vi "_FPGA_EventHandler.vi"(0 "LoadNextEvent_strobe":bool=TRUE, 7 "Reset_strobe":bool) -> (10 "Index+1?":u8, 12 "End?":bool, 13 "NewEvent_strobe?":bool, 14 "EventCode":u8, 15 "Param 1":u64, 16 "Param 2":u64, 17 "Param 3":u64, 18 "Param 4":u64, 19 "Param 5":u64)   [LabVIEW 2018]
uses:
  <instrlib>/_niInstr/Basic Elements/v1/FPGA/niInstr Basic Elements v1 FPGA.lvlib
  <instrlib>/_niInstr/Basic Elements/v1/FPGA/Private/Count Up U8.vi
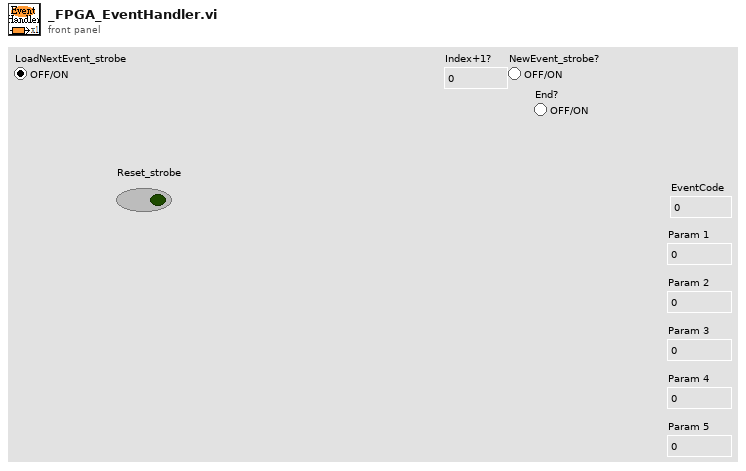
[diagram p1: front panel]
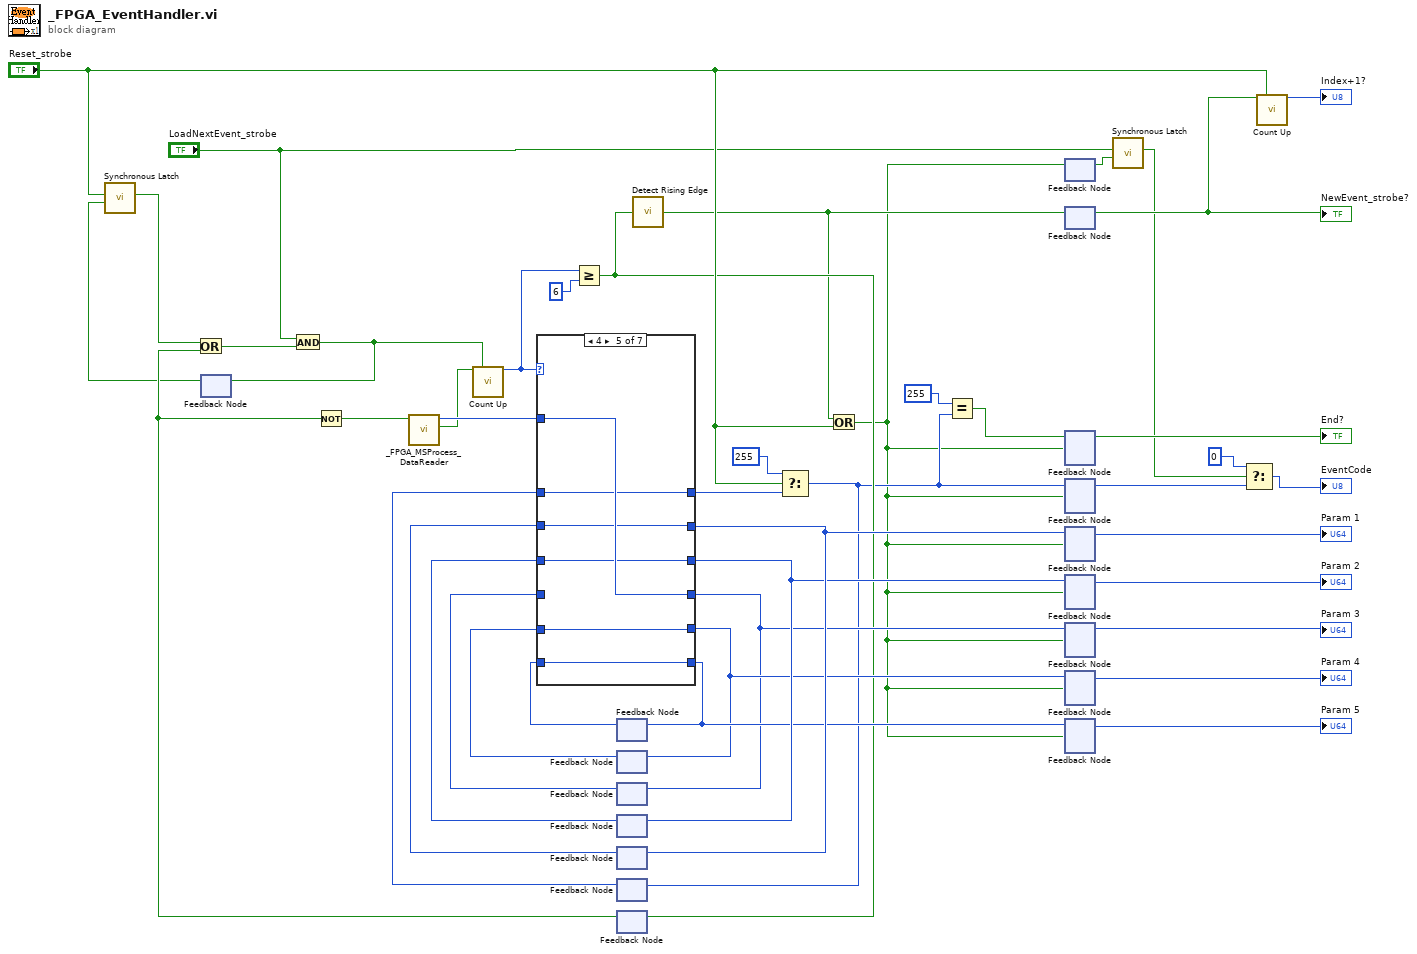
[diagram p0: block diagram]
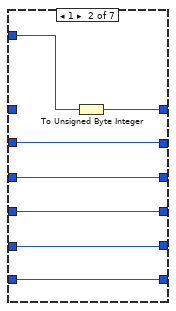
[diagram p3: hidden frame]
diagram:
  n1 = feedback #1() -> (w15:bool)  [unwired: 1 in]
  n2 = call <instrlib>:"Synchronous Latch.vi"("clear"=w15, "set"="Reset_strobe") -> ("out"=w14:bool)  [unwired: 9 in]
  n3 = feedback #2() -> (w41:u64)  [unwired: 1 in]
  n4 = feedback #3() -> (w40:u64)  [unwired: 1 in]
  n5 = feedback #4() -> (w39:u64)  [unwired: 1 in]
  n6 = feedback #5() -> (w32:u64)  [unwired: 1 in]
  n7 = feedback #6() -> (w33:u64)  [unwired: 1 in]
  n8 = feedback #7() -> (w34:u8)  [unwired: 1 in]
  n9 = feedback #8() -> (w20:bool)  [unwired: 1 in]
  n10 = Or(x=w14, y=w20) -> (x .or. y?=w16:bool)
  n11 = And(x="LoadNextEvent_strobe", y=w16) -> (x .and. y?=w8:bool)
  n12 = feedback-in #1(w8) -> ()
  n13 = Not(x=w20) -> (.not. x?=w36:bool)
  n14 = call "_FPGA_MSProcess_DataReader.vi"("Read"=w36) -> ("new value"=w42:bool, "Element"=w43:u64)  [unwired: 9 in]
  n15 = call-poly <instrlib>:"Count Up.vi"("increment"=w42, "reset"=w8) -> ("count out"=w38:u8)  [unwired: 13 in]
  n16 = case shown="4" w38 {
    tunnel: w43 -> [_ w57 w63 w69 w75 w81 w87]
    tunnel: [w45 w56 w62 w68 w74 w80 w86] -> w13
    tunnel: [w50 w55 w63 w67 w73 w79 w85] -> w31
    tunnel: [w49 w54 w61 w69 w72 w78 w84] -> w30
    tunnel: [w48 w53 w60 w66 w75 w77 w83] -> w27
    tunnel: [w47 w52 w59 w65 w71 w81 w82] -> w28
    tunnel: [w46 w51 w58 w64 w70 w76 w87] -> w29
    tunnel: w41 -> [w46 w51 w58 w64 w70 w76 _]
    tunnel: w40 -> [w47 w52 w59 w65 w71 _ w82]
    tunnel: w39 -> [w48 w53 w60 w66 _ w77 w83]
    tunnel: w32 -> [w49 w54 w61 _ w72 w78 w84]
    tunnel: w33 -> [w50 w55 _ w67 w73 w79 w85]
    tunnel: w34 -> [w45 _ w62 w68 w74 w80 w86]
    frame 0, Default {
    }
    frame 1 {
      n17 = To Unsigned Byte Integer(number=w57) -> (unsigned 8bit integer=w56:u8)
    }
    frame 2 {
    }
    frame 3 {
    }
    frame 4 {
    }
    frame 5 {
    }
    frame 6 {
    }
  }
  n18 = Greater Or Equal?(x=w38, y=u8 6) -> (x >= y?=w21:bool)
  n19 = feedback-in #2(w29) -> ()
  n20 = feedback-in #3(w28) -> ()
  n21 = feedback-in #4(w27) -> ()
  n22 = feedback-in #5(w30) -> ()
  n23 = feedback-in #6(w31) -> ()
  n24 = feedback-in #8(w21) -> ()
  n25 = call <instrlib>:"Detect Rising Edge.vi"("signal"=w21) -> ("edge detected"=w10:bool)  [unwired: 14 in]
  n26 = Select(t=u8 255, s="Reset_strobe", f=w13) -> (s? t:f=w11:u8)
  n27 = feedback-in #7(w11) -> ()
  n28 = Or(x=w10, y="Reset_strobe") -> (x .or. y?=w2:bool)
  n29 = Equal?(x=u8 255, y=w11) -> (x = y?=w9:bool)
  n30 = feedback #9() -> (w1:bool)  [unwired: 1 in]
  n31 = feedback-in #9(w2) -> ()
  n32 = feedback #10() -> (w6:bool)  [unwired: 1 in]
  "NewEvent_strobe?" <- w6
  n33 = feedback-in #10(w10) -> ()
  n34 = feedback #11() -> (→"End?":bool)  [unwired: 1 in]
  n35 = feedback-in #11(w9, w2) -> ()
  n36 = feedback-in #12(w11, w2) -> ()
  n37 = feedback #12() -> (w19:u8)  [unwired: 1 in]
  n38 = feedback #13() -> (→"Param 1":u64)  [unwired: 1 in]
  n39 = feedback-in #13(w31, w2) -> ()
  n40 = feedback #14() -> (→"Param 2":u64)  [unwired: 1 in]
  n41 = feedback-in #14(w30, w2) -> ()
  n42 = feedback #15() -> (→"Param 3":u64)  [unwired: 1 in]
  n43 = feedback-in #15(w27, w2) -> ()
  n44 = feedback #16() -> (→"Param 4":u64)  [unwired: 1 in]
  n45 = feedback-in #16(w28, w2) -> ()
  n46 = feedback #17() -> (→"Param 5":u64)  [unwired: 1 in]
  n47 = feedback-in #17(w29, w2) -> ()
  n48 = call <instrlib>:"Synchronous Latch.vi"("clear"=w1, "set"="LoadNextEvent_strobe") -> ("out"=w4:bool)  [unwired: 9 in]
  n49 = Select(t=u8 0, s=w4, f=w19) -> (s? t:f=→"EventCode":u8)
  n50 = call-poly <instrlib>:"Count Up.vi"("increment"=w6, "reset"="Reset_strobe") -> ("count out"=→"Index+1?":u8)  [unwired: 13 in]
